vi "Read_Camera.vi"(2 "node":string, 3 "Camera":T3, 4 "previous \nmage data":T1, 6 "error in":errorcluster) -> (0 "ROS Image":T2, 1 "image data":T1, 5 "error out":errorcluster)   [LabVIEW 2015]
doc: "Get an image from one of Baxter's hand cameras. \n\nIf you are running 1.1.0 or higher and reading an image in from the head camera, you must first close a hand camera and then open the head camera, waiting 5 s for each process to run.\n\nIt is highly recommended that you are connected to baxter via ethernet rather than over wireless when doing this."
uses:
  ROS/Code/SubVIs/BaxterCamera.ctl
  vi.lib/picture/picture.llb/imagedata.ctl
  ROS/Code/Console/Servers/ServerSubs/TopicDef.ctl
  ROS/Code/SubVIs/_ROSDirection.ctl
panel:
  out "image":picture
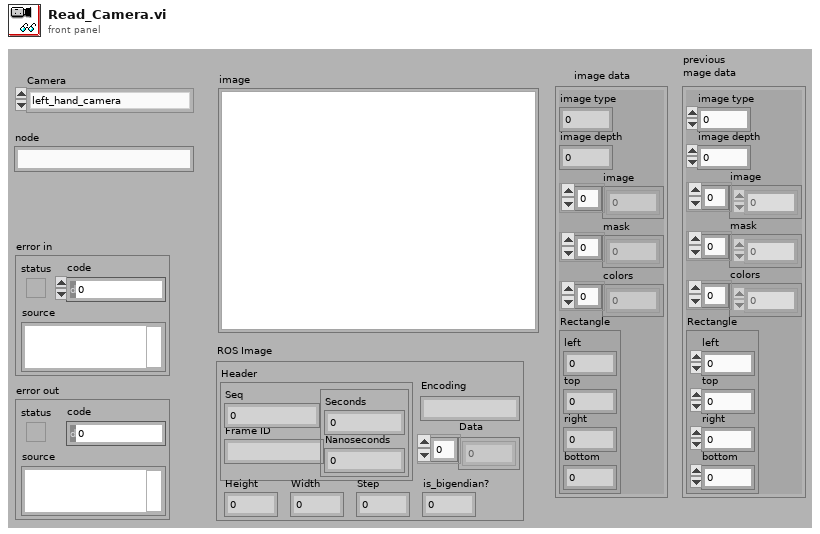
[diagram p1: front panel]
types:
  T1 = typedef "imagedata.ctl" = cluster{"image type":i32, "image depth":i32, "image":u8[], "mask":u8[], "colors":u32[], "Rectangle":cluster{"left":i16, "top":i16, "right":i16, "bottom":i16}}
  T2 = cluster{"Header":cluster{"Seq":u32, "Frame ID":string, cluster{"Seconds":i32, "Nanoseconds":i32}}, "Height":u32, "Width":u32, "is_bigendian?":u8, "Step":u32, "Data":u8[], "Encoding":string}
  T3 = typedef "BaxterCamera.ctl" = enum16{"left_hand_camera", "right_hand_camera", "head_camera"}
  T4 = typedef "TopicDef.ctl" = cluster{"Topic":string, "Type":string, "Action":T5, "Update (ms)":u16, "queue size":u16}
  T5 = typedef "_ROSDirection.ctl" = enum16{"Node", "Publisher", "Subscriber", "ServiceClient", "ServiceProvider"}
  T6 = typedef "_ROSControl.ctl" = cluster{"topic port":u16, "Node":string, "topic":string, "type":string, "node port":u16, "error ":errorcluster, "Direction":T5, "Update (ms)":u16, "FIFO size":u16}
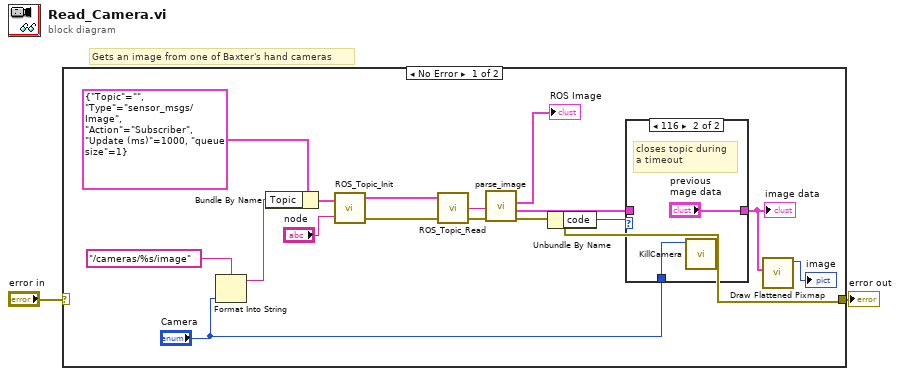
[diagram p0: block diagram]
diagram:
  # "Gets an image from one of Baxter's hand cameras"
  n1 = case shown="No Error" "error in" {
    selector: "error in" -> [_ w22]
    tunnel: [w4 w22] -> w2
    frame No Error {
      n2 = Format Into String(format string="/cameras/%s/image" ("topic"), "Camera") -> (resulting string=w14:string)  [unwired: 2 in, 1 out]
      n3 = Bundle By Name(cluster=T4 {"Topic"="", "Type"="sensor_msgs/Image", "Action"=enum."Subscriber", "Update (ms)"=1000, "queue size"=1} ("Definitions"), "Topic"=w14) -> (w13:T4)
      n4 = call "ROS_Topic_Init.vi"("Definitions"=w13, "node"="node") -> ("ROS out"=w17:T6, "error out"=w10:errorcluster)  [unwired: 1 in]
      n5 = call "ROS_Topic_Read.vi"("error in (no error)"=w10, "ROS in"=w17) -> ("error out"=w8:errorcluster, "Reply"=w9:string)  [unwired: 1 in, 1 out]
      n6 = call "parse_image.vi"("error in"=w8, "msg in"=w9) -> ("error out"=w4:errorcluster, "image data"=w6:T1, "ROS Image"=→"ROS Image":T2)  [unwired: 2 in, 1 out]
      n7 = Unbundle By Name(w4) -> ("code"=w3:i32)
      n8 = case shown="116" w3 {
        tunnel: "Camera" -> [_ w21]
        tunnel: w6 -> [w19 _]
        tunnel: [w19 "previous \nmage data"] -> w5
        frame Default {
        }
        frame 116 {
          # "closes topic during\na timeout"
          n9 = call "KillCamera.vi"("Camera"=w21) -> ()  [unwired: 11 in]
        }
      }
      "image data" <- w5
      n10 = call "Draw Flattened Pixmap.vi"("image data"=w5) -> ("new picture"=→"image":picture)  [unwired: 8 in]
    }
    frame Error {
    }
  }
  "error out" <- w2
